vi "写入.vi"(4 "测试人员":string, 6 "样品标记":string[](array[string]), 8 "error in (no error)":errorcluster, 11 "db file":path=path "D:/Data/样品标记.sqlite3") -> (0 "error out":errorcluster)   [LabVIEW 2020]
uses:
  <vilib>/drjdpowell/SQLite Library/SQL Statement/SQL Statement.lvclass/SQL Statement.ctl
  <vilib>/drjdpowell/SQLite Library/SQL Connection/Open (path).vi
  <vilib>/drjdpowell/SQLite Library/SQL Statement/Bind Text.vi
  <vilib>/drjdpowell/SQLite Library/SQL Connection/Open (string).vi
  <vilib>/drjdpowell/SQLite Library/SQL Statement/Step.vi
  <vilib>/AdvancedString/Path To Command Line String.vi
  <vilib>/drjdpowell/SQLite Library/SQL Connection/Execute SQL (No results).vi
  <vilib>/drjdpowell/SQLite Library/SQL Statement/Error Message.vi
  <vilib>/drjdpowell/SQLite Library/SQL Connection/Connection.lvclass
  <vilib>/drjdpowell/SQLite Library/SQL Statement/SQL Statement.lvclass
  <vilib>/drjdpowell/SQLite Library/Transaction Helpers/Transaction.lvlib
  <vilib>/drjdpowell/SQLite Library/SQLite.lvlib
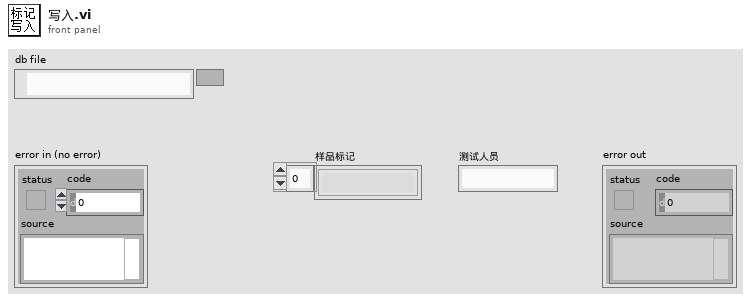
[diagram p1: front panel]
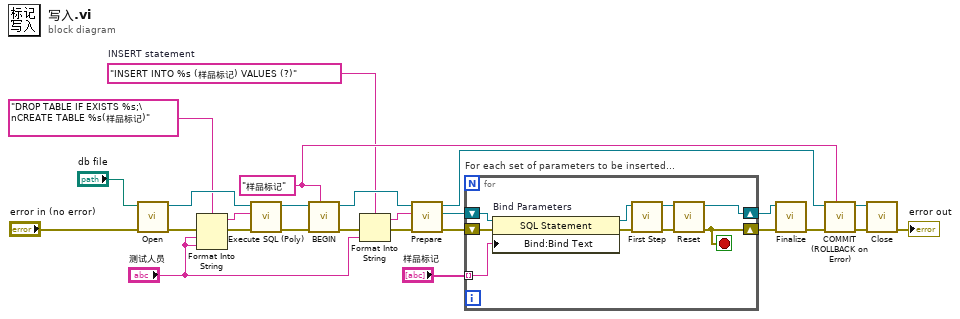
[diagram p0: block diagram]
diagram:
  w24 = "样品标记" ("Savepoint name")
  w20 = "INSERT INTO %s (样品标记) VALUES (?)"  # INSERT statement
  n1 = call-poly <vilib>:"Open.vi"("error in (no error)"="error in (no error)", "db file"="db file") -> ("error out"=w8:errorcluster, "SQLite Connection"=w15:refnum<class "Connection.lvclass">)  [unwired: 8 in]
  n2 = Format Into String(format string="DROP TABLE IF EXISTS %s;\nCREATE TABLE %s(样品标记)" ("SQL"), error in=w8, "测试人员", "测试人员") -> (resulting string=w9:string, error out=w7:errorcluster)  [unwired: 1 in]
  n3 = call-poly <vilib>:"Execute SQL (Poly).vi"("error in (no error)"=w7, "SQL"=w9, "SQLite Connection in"=w15) -> ("error out"=w12:errorcluster, "SQLite Connection"=w17:refnum<class "Connection.lvclass">)  [unwired: 7 in]
  n4 = call <vilib>:"BEGIN.vi"("Savepoint name"=w24, "error in (no error)"=w12, "SQLite Connection in"=w17) -> ("error out"=w5:errorcluster, "SQLite Connection"=w23:refnum<class "Connection.lvclass">)  [unwired: 7 in]
  n5 = Format Into String(format string=w20, error in=w5, "测试人员") -> (resulting string=w10:string, error out=w4:errorcluster)  [unwired: 1 in]
  n6 = call <vilib>:"Prepare.vi"("error in (no error)"=w4, "SQL"=w10, "SQLite Connection in"=w23) -> ("error out"=w19:errorcluster, "SQL Statement"=w18:refnum<class "SQL Statement.lvclass">, "SQLite Connection"=w25:refnum<class "Connection.lvclass">)  [unwired: 4 in, 2 out]
  n7 = for "For each set of parameters to be inserted..." {
    shift-right: [w29] -> w21
    shift-left: w18 -> [w35]
    shift-right: [w28] -> w22
    shift-left: w19 -> [w32]
    tunnel: "样品标记" -> [w27] mode=indexing
    stop <- w28 stop-if-true
    n8 = property on="Bind Parameters" class="SQL Statement"(reference=w35, error in=w32, "Bind:Bind Text"=w27) -> (reference out=w34:refnum<class "SQL Statement.lvclass">, error out=w33:errorcluster)
    n9 = call <vilib>:"First Step.vi"("error in (no error)"=w33, "SQL Statement in"=w34) -> ("error out"=w31:errorcluster, "SQL Statement"=w30:refnum<class "SQL Statement.lvclass">)  [unwired: 7 in, 1 out]
    n10 = call <vilib>:"Reset.vi"("error in (no error)"=w31, "SQL Statement in"=w30) -> ("error out"=w28:errorcluster, "SQL Statement"=w29:refnum<class "SQL Statement.lvclass">)  [unwired: 8 in]
  }
  n11 = call <vilib>:"Finalize.vi"("error in (no error)"=w22, "SQL Statement in"=w21) -> ("error out"=w26:errorcluster)  [unwired: 9 in]
  n12 = call <vilib>:"COMMIT (ROLLBACK on Error).vi"("Savepoint name"=w24, "error in (no error)"=w26, "SQLite Connection in"=w25) -> ("error out"=w6:errorcluster, "SQLite Connection"=w16:refnum<class "Connection.lvclass">)  [unwired: 7 in]
  n13 = call-dynamic "Close.vi"("error in (no error)"=w6, "SQLite Connection in"=w16) -> ("error out"=→"error out":errorcluster)  [unwired: 9 in]
